vi "set_I_channel.vi"(8 "error in (no error)":errorcluster, 9 "current":dbl min=0.0 max=5.0, 10 "channel":T1=enum."1", 11 "DC_power_supply in":refnum<class "DC_power_supply.lvclass">) -> (0 "error out":errorcluster, 3 "DC_power_supply out":refnum<class "DC_power_supply.lvclass">)   [LabVIEW 2017, in "DC_power_supply.lvclass"]
uses:
  DC_power_supply.lvclass
  subVI/motech_power_supply/types/channels_enum.ctl
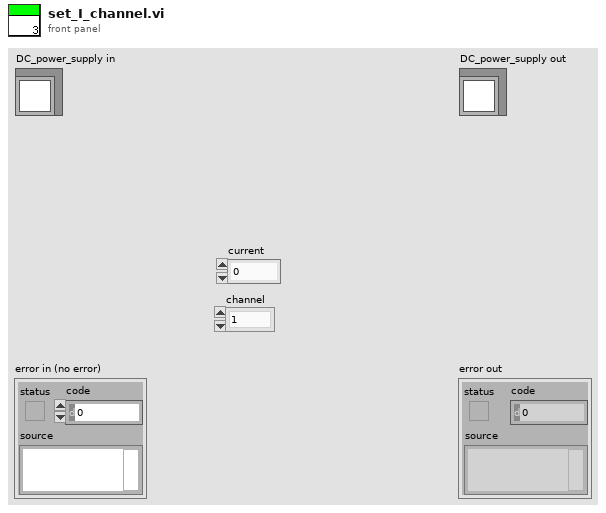
[diagram p1: front panel]
types:
  T1 = typedef "channels_enum.ctl" = enum16{"0", "1", "2"}
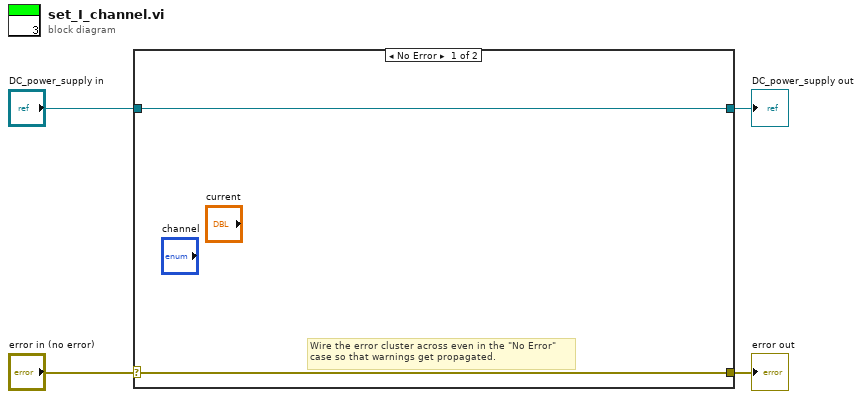
[diagram p0: block diagram]
diagram:
  n1 = case shown="No Error" "error in (no error)" {
    selector: "error in (no error)" -> [w5 w8]
    tunnel: [w5 w8] -> w3
    tunnel: [w6 w7] -> w1
    tunnel: "DC_power_supply in" -> [w6 w7]
    frame No Error {
      # "Wire the error cluster across even in the \"No Error\"\ncase so that warnings get propagated."
    }
    frame Error {
    }
  }
  "error out" <- w3
  "DC_power_supply out" <- w1
